vi "Change DAQ Rate.vi"(8 "error in (no error)":errorcluster, 11 "tCRD in":refnum<class "Aircraft OPCCRD.lvclass">) -> (0 "error out":errorcluster, 3 "tCRD out":refnum<class "Aircraft OPCCRD.lvclass">)   [LabVIEW 2015, in "Aircraft OPCCRD.lvclass"]
uses:
  Aircraft OPCCRD.lvclass
  FPGA/Rate.ctl
  Reusable/Instrument/Instrument.lvclass/Instrument.ctl
  Aircraft OPCCRD.lvclass/Aircraft OPCCRD.ctl
  Reusable/Instrument/Read Log Session.vi
  Accessors/Read FPGA Ref.vi
  Accessors/Write SamplesPerRep.vi
  Reusable/CRDS/Main/Read Cells.vi
  <vilib>/Utility/error.llb/Error Cluster From Error Code.vi
  <vilib>/rvi/errors/niLvFpgaAdjustHostInterfaceError.vi
  Reusable/CRDS/Cell/Write dt.vi
  Reusable/CRDS/Main/Write Cells.vi
  <userlib>/_Session Fwk/Session - Root.lvclass
  tFPGA Ref.ctl
  Reusable/CRDS/Cell/CRDS Cell.lvclass
  <vilib>/rvi/interface/nirviReadWriteControl/nirviReadWriteControl.xnode
  FPGA Bitfiles/Aircraft OPCRD Server.lvbitx
  Reusable/Instrument/Instrument.lvclass
  Reusable/Session Log/System Log.lvclass
  NiFpgaLv.dll
panel:
  out "rate":T1 items=["1 MHz"=20, "2 MHz"=10, "2.5 MHz"=8, "5 MHz"=4, "10 MHz"=2, "20MHz"=1]
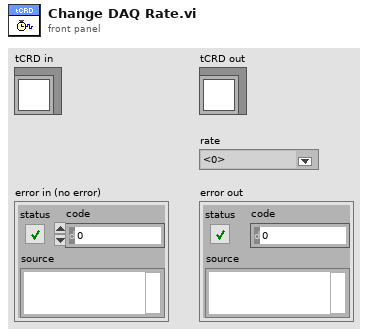
[diagram p1: front panel]
types:
  T1 = typedef "Rate.ctl" = u8
  T2 = typedef "Session - Root.lvclass/Session Handle.ctl" = refnum<data-value>
  T3 = typedef "Aircraft OPCCRD.lvclass/tFPGA Ref.ctl" = refnum<k20>
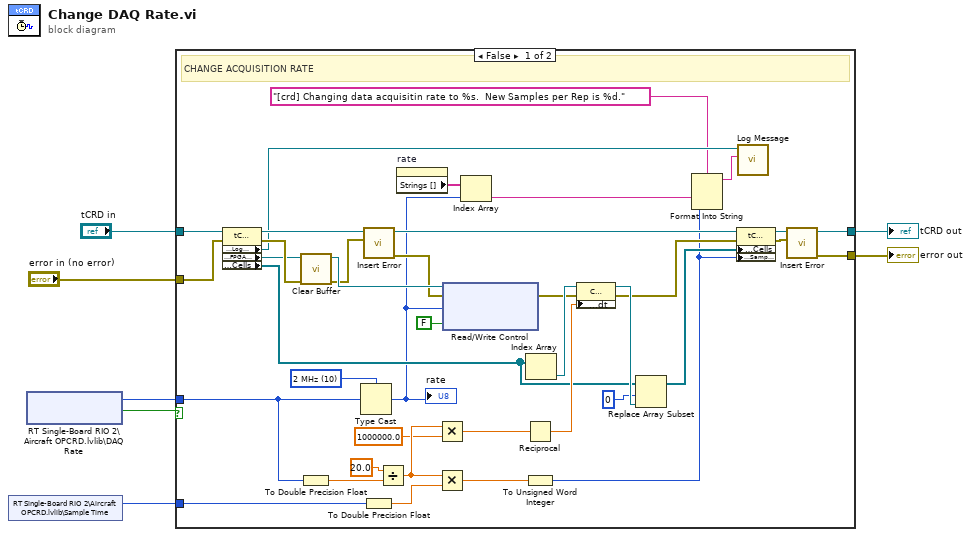
[diagram p0: block diagram]
diagram:
  n1 = shared-variable "RT Single-Board RIO 2\\Aircraft OPCRD.lvlib\\Sample Time"() -> (w7:u16)  [unwired: 1 in, 1 out]
  n2 = shared-variable "RT Single-Board RIO 2\\Aircraft OPCRD.lvlib\\DAQ Rate"() -> (w2:u8, w3:bool)  [unwired: 2 in, 1 out]
  n3 = case shown="False" w3 {
    tunnel: "error in (no error)" -> [w26 w48]
    tunnel: "tCRD in" -> [w35 w47]
    tunnel: w2 -> [w19 _]
    tunnel: [w18 w48] -> w6
    tunnel: [w22 w47] -> w5
    tunnel: w7 -> [w29 _]
    frame False {
      w20 = T1 10 items=["1 MHz"=20, "2 MHz"=10, "2.5 MHz"=8, "5 MHz"=4, "10 MHz"=2, "20MHz"=1] ("Rate")
      # "CHANGE ACQUISITION RATE"
      n4 = property class="tCRD"(reference=w35, error in=w26) -> (reference out=w25:refnum<class "Aircraft OPCCRD.lvclass">, error out=w34:errorcluster, "Accessors:Log Session"=w14:T2, "Accessors:FPGA Ref"=w15:T3, "Data Access:Cells"=w32:refnum<class "CRDS Cell.lvclass">[])
      n5 = call "Clear Buffer.vi"("error in"=w34, "Refnum in"=w15) -> ("error out"=w24:errorcluster, "FPGA VI Reference Out"=w33:T3)  [unwired: 8 in]
      n6 = To Double Precision Float(number=w19) -> (double precision float=w30:dbl)
      n7 = Type Cast(type=w20, x=w19) -> (*(type *) &x=w12:T1)
      "rate" <- w12
      n8 = call "Insert Error.vi"("err"=w24, "Instrument in"=w25) -> ("error out"=w23:errorcluster, "Instrument out"=w21:refnum<class "Aircraft OPCCRD.lvclass">)  [unwired: 7 in, 1 out]
      n9 = To Double Precision Float(number=w29) -> (double precision float=w28:dbl)
      n10 = Divide(x=20.0, y=w30) -> (x/y=w42:dbl)
      n11 = property on="rate" class="Ring (strict)"() -> ("Strings []"=w11:string[])  [unwired: 2 in, 2 out]
      n12 = Multiply(x=w42, y=1000000.0) -> (x*y=w40:dbl)
      n13 = Multiply(x=w42, y=w28) -> (x*y=w44:dbl)
      n14 = xnode "Read/Write Control"("FPGA VI Reference In"=w33, "error in"=w23, "Rate"=w12, "Pause Digitizer"=FALSE) -> ("error out"=w31:errorcluster)  [unwired: 1 out]
      n15 = Index Array(array=w11, index=w12) -> (element=w10:string)
      n16 = Reciprocal(x=w40) -> (1/x=w39:dbl)
      n17 = To Unsigned Word Integer(number=w44) -> (unsigned 16bit integer=w9:u16)
      n18 = Index Array(array=w32) -> (element=w43:refnum<class "CRDS Cell.lvclass">)  [unwired: 1 in]
      n19 = property class="CRDS Cell"(reference=w43, error in=w31, "Data Access:dt"=w39) -> (reference out=w38:refnum<class "CRDS Cell.lvclass">, error out=w27:errorcluster)
      n20 = Replace Array Subset(array=w32, new element=w38, index=0) -> (w36:refnum<class "CRDS Cell.lvclass">[])
      n21 = Format Into String(format string="[crd] Changing data acquisitin rate to %s.  New Samples per Rep is %d." ("MSG In"), w10, w9) -> (resulting string=w8:string)  [unwired: 2 in, 1 out]
      n22 = property class="tCRD"(reference=w21, error in=w27, "Data Access:Cells"=w36, "Accessors:SamplesPerRep"=w9) -> (reference out=w17:refnum<class "Aircraft OPCCRD.lvclass">, error out=w16:errorcluster)
      n23 = call "Log Message.vi"("MSG In"=w8, "session in"=w14) -> ()  [unwired: 8 in, 2 out]
      n24 = call "Insert Error.vi"("err"=w16, "Instrument in"=w17) -> ("error out"=w18:errorcluster, "Instrument out"=w22:refnum<class "Aircraft OPCCRD.lvclass">)  [unwired: 7 in, 1 out]
    }
    frame True {
    }
  }
  "error out" <- w6
  "tCRD out" <- w5
